vi "Find_nb_of_occurence_in_str.vi"(2 "search string/char":string, 3 "Str In":string) -> (0 "Index":i32, 1 "Nb of occurrence":i32)   [LabVIEW 2011]
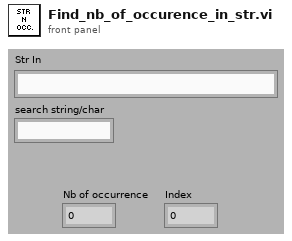
[diagram p1: front panel]
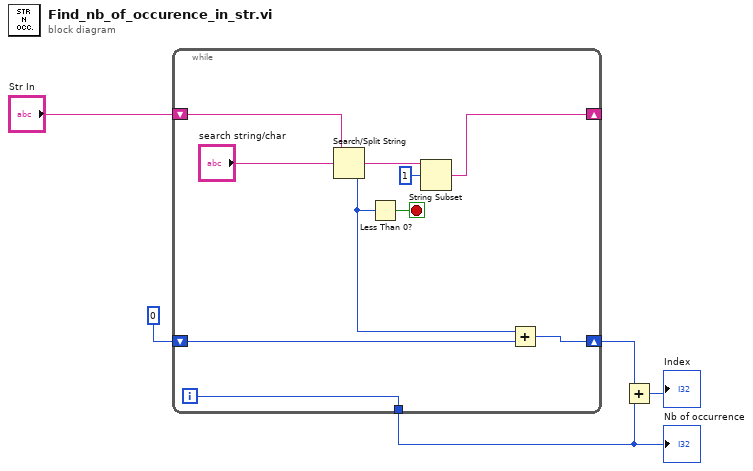
[diagram p0: block diagram]
diagram:
  n1 = while {
    shift-right: [w12] -> _
    shift-left: "Str In" -> [w15]
    tunnel: [w10] -> w1
    shift-right: [w8] -> w2
    shift-left: 0 ("Index") -> [w7]
    i -> [w10]
    stop <- w11 stop-if-true
    n2 = Search/Split String(string=w15, search string/char (-)="search string/char") -> (match + rest of string=w14:string, offset of match=w6:i32)  [unwired: 1 in, 1 out]
    n3 = Less Than 0?(x=w6) -> (x < 0?=w11:bool)
    n4 = String Subset(string=w14, offset (0)=1) -> (substring=w12:string)  [unwired: 1 in]
    n5 = Add(x=w6, y=w7) -> (x+y=w8:i32)
  }
  "Nb of occurrence" <- w1
  n6 = Add(x=w2, y=w1) -> (x+y=→"Index":i32)
